vi "EST.Input.Generate.vi"(8 "error in (no error)":errorcluster, 11 "Parameters":T1) -> (0 "error out":errorcluster)   [LabVIEW 2015]
uses:
  EST.Inputs.Generate.Parameters.ctl
  <vilib>/Utility/miscctls.llb/LVPointTypeDef.ctl
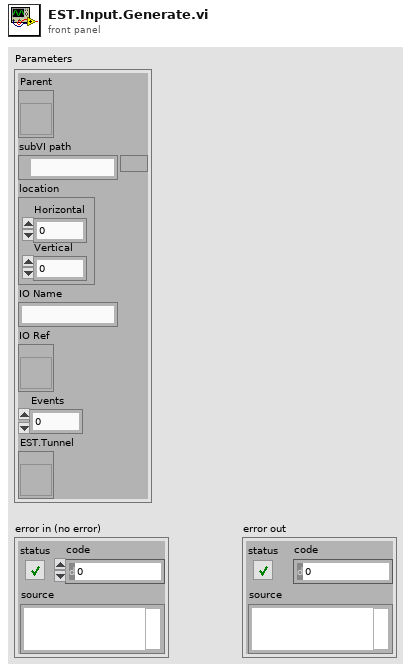
[diagram p1: front panel]
types:
  T1 = typedef "EST.Inputs.Generate.Parameters.ctl" = cluster{"Parent":refnum<vi>, "subVI path":path, "location":T2, "IO Name":string, "IO Ref":refnum<vi>, "Events":u32, "EST.Tunnel":refnum<vi>}
  T2 = typedef "LVPointTypeDef.ctl" = cluster{"Horizontal":i16, "Vertical":i16}
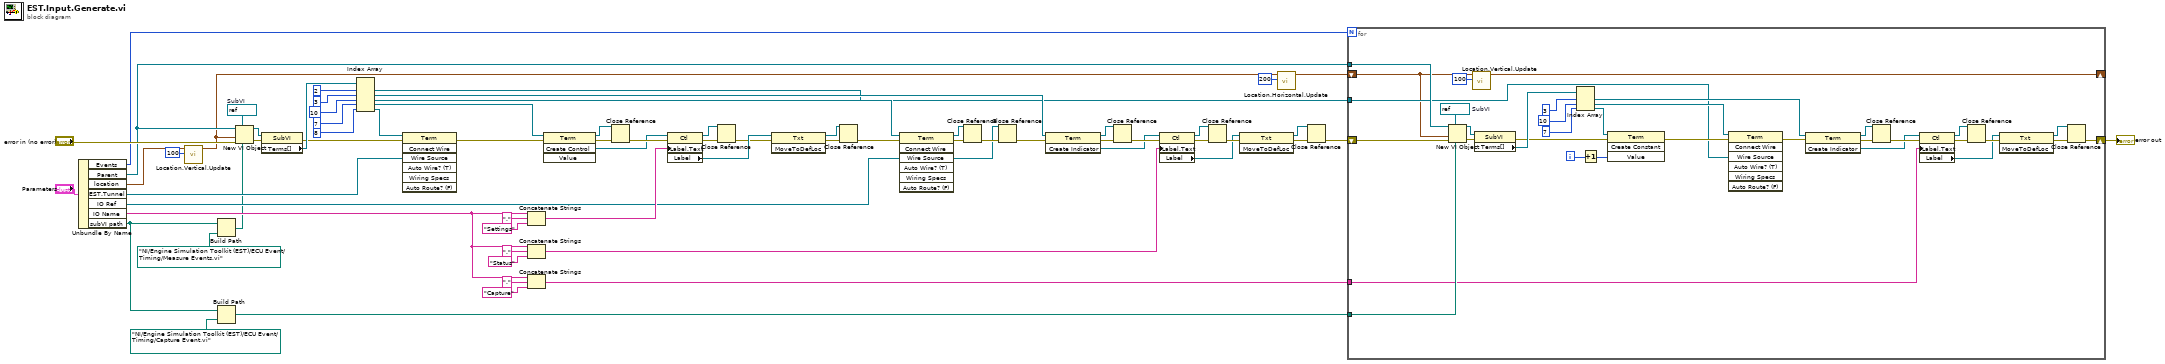
[diagram p0: block diagram]
diagram:
  w47 = refnum<vi> refnum  # SubVI
  n1 = Unbundle By Name("Parameters") -> ("Events"=w23:u32, "Parent"=w22:refnum<vi>, "location"=w14:T2, "EST.Tunnel"=w6:refnum<vi>, "IO Ref"=w45:refnum<vi>, "IO Name"=w17:string, "subVI path"=w1:path)
  n2 = call "Location.Vertical.Update.vi"("Vertical Change"=i16 100, "location in"=w14) -> ("location out"=w12:T2)  [unwired: 9 in]
  n3 = Build Path(base path=w1, name or relative path=path "NI/Engine Simulation Toolkit (EST)/ECU Event/Timing/Measure Events.vi" ("path")) -> (appended path=w4:path)
  n4 = Build Path(base path=w1, name or relative path=path "NI/Engine Simulation Toolkit (EST)/ECU Event/Timing/Capture Event.vi" ("path")) -> (appended path=w2:path)
  n5 = New VI Object(vi object class=w47, owner refnum=w22, position/next to=w12, 6:w4, 8:"error in (no error)") -> (object refnum=w50:refnum<vi>, 0:w51:errorcluster)  [unwired: 3 in]
  n6 = property class="SubVI"(reference=w50, error in=w51) -> (error out=w8:errorcluster, "Terms[]"=w49:refnum<vi>[])  [unwired: 1 out]
  n7 = Index Array(array=w49, index #1=2 ("index"), index #2=3 ("index"), index #3=10 ("index"), index #4=7 ("index"), index #5=8 ("index")) -> (element #1=w20:refnum<vi>, element #2=w26:refnum<vi>, element #3=w27:refnum<vi>, element #4=w28:refnum<vi>, element #5=w9:refnum<vi>)
  n8 = invoke class="Term" method="Connect Wire"(reference=w9, error in=w8, "Wire Source"=w6) -> (error out=w7:errorcluster)  [unwired: 4 in, 6 out]
  n9 = Concatenate Strings(w17, "." ("string"), "Settings" ("string")) -> (w52:string)
  n10 = Concatenate Strings(w17, "." ("string"), "Status" ("string")) -> (w21:string)
  n11 = Concatenate Strings(w17, "." ("string"), "Capture" ("string")) -> (w16:string)
  n12 = invoke class="Term" method="Create Control"(reference=w28, error in=w7) -> (reference out=w59:refnum<vi>, error out=w58:errorcluster, "Create Control"=w44:refnum<vi>)  [unwired: 2 in, 1 out]
  n13 = Close Reference(reference=w59, error in (no error)=w58) -> (error out=w60:errorcluster)
  n14 = property class="Ctl"(reference=w44, error in=w60, "Label.Text"=w52) -> (reference out=w43:refnum<vi>, error out=w41:errorcluster, "Label"=w42:refnum<vi>)
  n15 = Close Reference(reference=w43, error in (no error)=w41) -> (error out=w40:errorcluster)
  n16 = invoke class="Txt" method="MoveToDefLoc"(reference=w42, error in=w40) -> (reference out=w38:refnum<vi>, error out=w39:errorcluster)  [unwired: 1 in, 1 out]
  n17 = Close Reference(reference=w38, error in (no error)=w39) -> (error out=w37:errorcluster)
  n18 = invoke class="Term" method="Connect Wire"(reference=w27, error in=w37, "Wire Source"=w45) -> (reference out=w62:refnum<vi>, error out=w61:errorcluster)  [unwired: 4 in, 5 out]
  n19 = Close Reference(reference=w62, error in (no error)=w61) -> (error out=w63:errorcluster)
  n20 = Close Reference(reference=w45, error in (no error)=w63) -> (error out=w64:errorcluster)
  n21 = invoke class="Term" method="Create Indicator"(reference=w26, error in=w64) -> (reference out=w67:refnum<vi>, error out=w68:errorcluster, "Create Indicator"=w55:refnum<vi>)  [unwired: 1 in]
  n22 = Close Reference(reference=w67, error in (no error)=w68) -> (error out=w69:errorcluster)
  n23 = property class="Ctl"(reference=w55, error in=w69, "Label.Text"=w21) -> (reference out=w65:refnum<vi>, error out=w66:errorcluster, "Label"=w34:refnum<vi>)
  n24 = Close Reference(reference=w65, error in (no error)=w66) -> (error out=w35:errorcluster)
  n25 = invoke class="Txt" method="MoveToDefLoc"(reference=w34, error in=w35) -> (reference out=w33:refnum<vi>, error out=w36:errorcluster)  [unwired: 1 in, 1 out]
  n26 = call "Location.Horizontal.Update.vi"("Horizontal Change"=i16 200 ("Vertical Change"), "location in"=w12) -> ("location out"=w11:T2)  [unwired: 9 in]
  n27 = Close Reference(reference=w33, error in (no error)=w36) -> (error out=w25:errorcluster)
  n28 = for {
    N: w23 -> [_]
    shift-right: [w82] -> w24
    shift-left: w25 -> [w100]
    tunnel: w22 -> [w99]
    tunnel: w2 -> [w98]
    tunnel: w16 -> [w81]
    tunnel: w20 -> [w73]
    shift-right: [w70] -> _
    shift-left: w11 -> [w71]
    i -> [w78]
    w101 = refnum<vi> refnum  # SubVI
    n29 = New VI Object(vi object class=w101, owner refnum=w99, position/next to=w71, 6:w98, 8:w100) -> (object refnum=w102:refnum<vi>, 0:w103:errorcluster)  [unwired: 3 in]
    n30 = call "Location.Vertical.Update.vi"("Vertical Change"=i16 100, "location in"=w71) -> ("location out"=w70:T2)  [unwired: 9 in]
    n31 = property class="SubVI"(reference=w102, error in=w103) -> (error out=w79:errorcluster, "Terms[]"=w97:refnum<vi>[])  [unwired: 1 out]
    n32 = Index Array(array=w97, index #1=3 ("index"), index #2=10 ("index"), index #3=7 ("index")) -> (element #1=w83:refnum<vi>, element #2=w76:refnum<vi>, element #3=w80:refnum<vi>)
    n33 = Increment(x=w78) -> (x+1=w77:i32)
    n34 = invoke class="Term" method="Create Constant"(reference=w80, error in=w79, "Value"=w77) -> (error out=w75:errorcluster)  [unwired: 1 in, 3 out]
    n35 = invoke class="Term" method="Connect Wire"(reference=w76, error in=w75, "Wire Source"=w73) -> (error out=w74:errorcluster)  [unwired: 4 in, 6 out]
    n36 = invoke class="Term" method="Create Indicator"(reference=w83, error in=w74) -> (reference out=w91:refnum<vi>, error out=w92:errorcluster, "Create Indicator"=w88:refnum<vi>)  [unwired: 1 in]
    n37 = Close Reference(reference=w91, error in (no error)=w92) -> (error out=w93:errorcluster)
    n38 = property class="Ctl"(reference=w88, error in=w93, "Label.Text"=w81) -> (reference out=w89:refnum<vi>, error out=w90:errorcluster, "Label"=w85:refnum<vi>)
    n39 = Close Reference(reference=w89, error in (no error)=w90) -> (error out=w86:errorcluster)
    n40 = invoke class="Txt" method="MoveToDefLoc"(reference=w85, error in=w86) -> (reference out=w84:refnum<vi>, error out=w87:errorcluster)  [unwired: 1 in, 1 out]
    n41 = Close Reference(reference=w84, error in (no error)=w87) -> (error out=w82:errorcluster)
  }
  "error out" <- w24
